vi "ConvertStringToFloat_Scalar.vi"(7 "default value (NaN)":dbl=nan format="%#_13g", 11 "String":string) -> (3 "Double":dbl, 5 "error out":errorcluster)   [LabVIEW 2022 SP3, in "hse-misc.lvlib"]
doc: "converts single string value to floating point value\n\n____\nHAMPEL SOFTWARE ENGINEERING v3.8.0 (2023-12-18 14:41)"
uses:
  hse-misc.lvlib
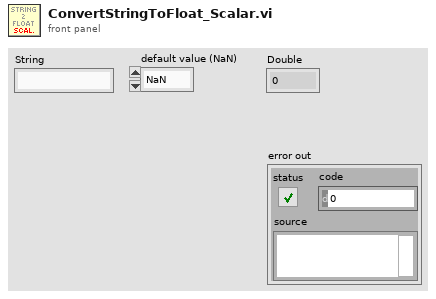
[diagram p1: front panel]
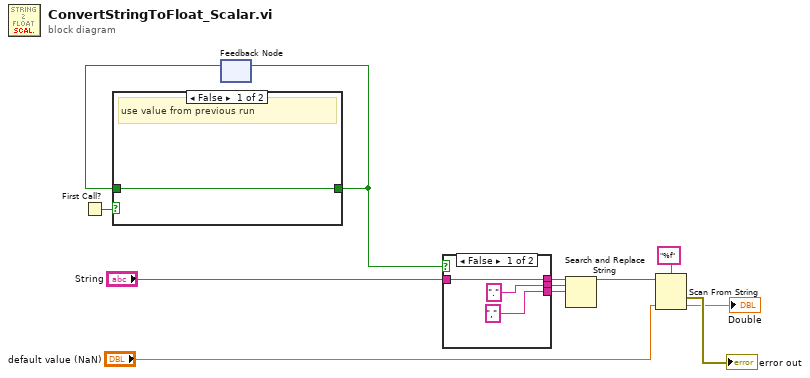
[diagram p0: block diagram]
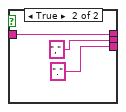
[diagram p2: hidden frame]
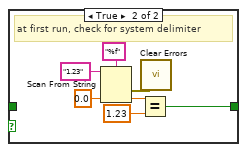
[diagram p3: hidden frame]
diagram:
  n1 = First Call?() -> (First Call?: T/F=w11:bool)
  n2 = feedback #1() -> (w4:bool)  [unwired: 1 in]
  n3 = case shown="False" w11 {
    tunnel: [w13 w14] -> w5
    tunnel: w4 -> [w13 _]
    frame False {
      # "use value from previous run"
    }
    frame True {
      # "at first run, check for system delimiter"
      n4 = Scan From String(format string="%f", input string="1.23", default 1=0.0 ("default value 1")) -> (error out=w18:errorcluster, output 1=w16:dbl)  [unwired: 2 in, 2 out]
      n5 = Equal?(x=w16, y=1.23) -> (x = y?=w14:bool)
      n6 = call <vilib>:"Clear Errors.vi"("error in (no error)"=w18) -> ()  [unwired: 5 in, 2 out]
    }
  }
  n7 = feedback-in #1(w5) -> ()
  n8 = case shown="False" w5 {
    tunnel: "String" -> [w23 w26]
    tunnel: [w23 w26] -> w10
    tunnel: ["." ("search string") "," ("search string")] -> w9
    tunnel: ["," ("replace string (\"\")") "." ("replace string (\"\")")] -> w8
    frame False {
    }
    frame True {
    }
  }
  n9 = Search and Replace String(input string=w10, search string=w9, replace string=w8) -> (result string=w7:string)  [unwired: 5 in, 3 out]
  n10 = Scan From String(format string="%f", input string=w7, default 1="default value (NaN)") -> (error out=→"error out":errorcluster, output 1=→"Double":dbl)  [unwired: 2 in, 2 out]
